vi "Main.vi"() -> ()   [LabVIEW 2013]
uses:
  <userlib>/KNR OS 3.0 LabVIEW Toolkit/Type Definition/Resource.ctl
panel:
  out "Numeric":i32
  out "LED List":bool[](array[boolean])
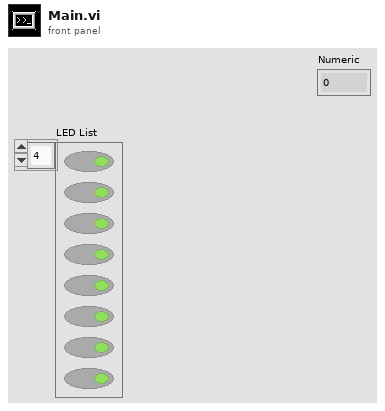
[diagram p1: front panel]
types:
  T1 = typedef "Resource.ctl" = enum16{"KNRm_DDRC", "KNRm_DDDD", "KNRm_DDDR", "KNRm_DDDC", "KNR"}
  T2 = typedef "KNR3 Reference.ctl" = cluster{"FPGA Session":refnum<class "FPGA Interface Base.lvclass">, "Resource":T1}
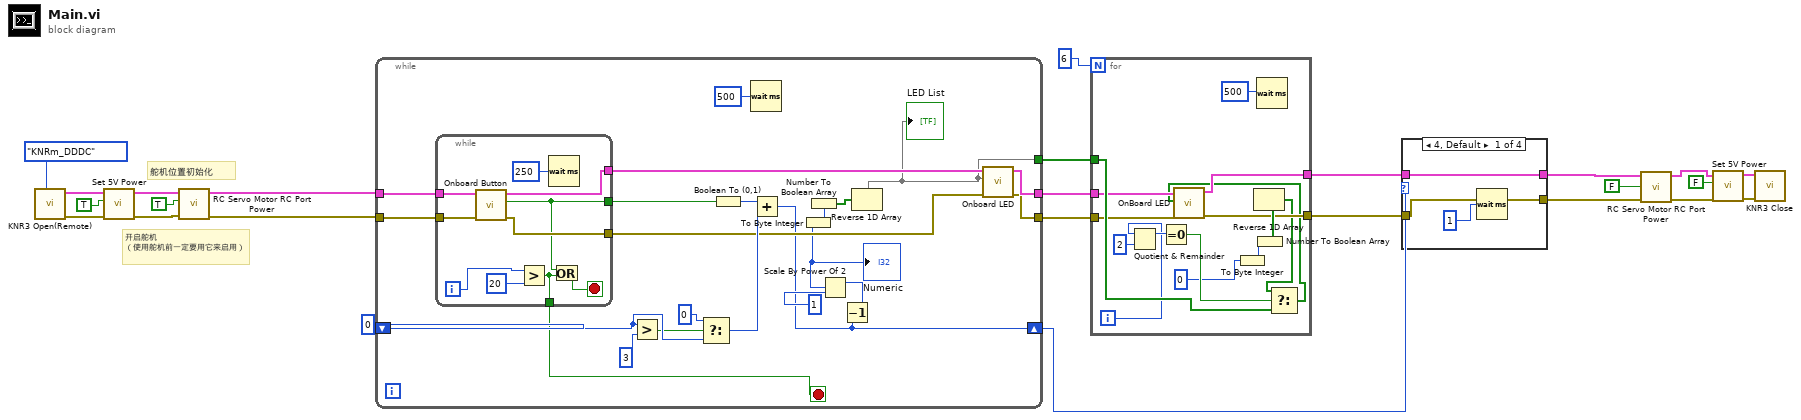
[diagram p0: block diagram]
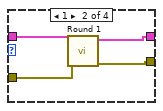
[diagram p2: hidden frame]
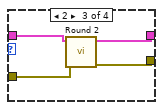
[diagram p3: hidden frame]
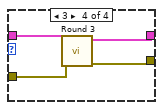
[diagram p4: hidden frame]
diagram:
  # "开启舵机\n（使用舵机前一定要用它来启用）"
  # "舵机位置初始化"
  n1 = call <userlib>:"KNR3 Open(Remote).vi"("Resource"=Resource."KNRm_DDDC") -> ("error out"=w22:errorcluster, "KNR out"=w23:T2)  [unwired: 9 in]
  n2 = call <userlib>:"Set 5V Power.vi"("error in (no error)"=w22, "5V Power(T)"=TRUE, "KNR in"=w23) -> ("error out"=w18:errorcluster, "KNR out"=w19:T2)  [unwired: 7 in]
  n3 = call <userlib>:"RC Servo Motor RC Port Power.vi"("error in (no error)"=w18, "RC Power(F)"=TRUE, "KNR in"=w19) -> ("error out"=w16:errorcluster, "KNR out"=w17:T2)  [unwired: 7 in]
  n4 = while {
    shift-right: [w30] -> w4
    shift-left: i8 0 -> [w46]
    tunnel: w17 -> [w42]
    tunnel: w16 -> [w41]
    tunnel: [w35] -> w3
    tunnel: [w34] -> w2
    tunnel: [w28] -> w1
    stop <- w27 stop-if-true
    n5 = while {
      tunnel: [w50] -> w44
      tunnel: w42 -> [w57]
      tunnel: w41 -> [w56]
      tunnel: [w54] -> w37
      tunnel: [w53] -> w36
      tunnel: [w48] -> w27
      i -> [w51]
      stop <- w49 stop-if-true
      n6 = call <userlib>:"Onboard Button.vi"("error in (no error)"=w56, "KNR in"=w57) -> ("error out"=w53:errorcluster, "value"=w50:bool, "KNR out"=w54:T2)  [unwired: 7 in]
      n7 = Greater?(x=w51, y=20) -> (0:w48:bool)
      n8 = Wait (ms)(milliseconds to wait=u32 250) -> ()  [unwired: 1 out]
      n9 = Or(x=w50, y=w48) -> (x .or. y?=w49:bool)
    }
    n10 = Greater?(x=w46, y=i8 3) -> (0:w39:bool)
    n11 = Select(t=0, s=w39, f=w46) -> (s? t:f=w45:i32)
    n12 = Boolean To (0,1)(Boolean=w44) -> (0, 1=w43:i16)
    n13 = Wait (ms)(milliseconds to wait=u32 500) -> ()  [unwired: 1 out]
    n14 = Add(x=w43, y=w45) -> (x+y=w30:i32)
    n15 = Decrement(x=w30) -> (x-1=w29:i32)
    n16 = Scale By Power Of 2(n=w29, x=1) -> (x*2^n=w32:i32)
    "Numeric" <- w32
    n17 = To Byte Integer(number=w32) -> (8bit integer=w31:i8)
    n18 = Number To Boolean Array(number=w31) -> (Boolean array=w38:bool[])
    n19 = Reverse 1D Array(array=w38) -> (reversed array=w28:bool[])
    "LED List" <- w28
    n20 = call <userlib>:"Onboard LED.vi"("error in (no error)"=w36, "LED List"=w28, "KNR in"=w37) -> ("error out"=w34:errorcluster, "KNR out"=w35:T2)  [unwired: 7 in]
  }
  n21 = for {
    N: i8 6 -> [_]
    tunnel: w1 -> [w70]
    tunnel: w3 -> [w66]
    tunnel: w2 -> [w65]
    tunnel: [w63] -> w7
    tunnel: [w62] -> w5
    i -> [w64]
    n22 = Quotient & Remainder(x=w64, y=i8 2) -> (x-y*floor(x/y)=w69:i32)  [unwired: 1 out]
    n23 = Equal To 0?(x=w69) -> (x = 0?=w68:bool)
    n24 = To Byte Integer(number=0) -> (8bit integer=w61:i8)
    n25 = Number To Boolean Array(number=w61) -> (Boolean array=w67:bool[])
    n26 = Reverse 1D Array(array=w67) -> (reversed array=w59:bool[])
    n27 = Wait (ms)(milliseconds to wait=500) -> ()  [unwired: 1 out]
    n28 = Select(t=w59, s=w68, f=w70) -> (s? t:f=w58:bool[])
    n29 = call <userlib>:"OnBoard LED.vi"("error in (no error)"=w65, "LED List"=w58, "KNR in"=w66) -> ("error out"=w62:errorcluster, "KNR out"=w63:T2)  [unwired: 7 in]
  }
  n30 = case shown="4, Default" w4 {
    tunnel: [w75 w77 w81 w86] -> w8
    tunnel: w7 -> [w75 w79 w83 w87]
    tunnel: [w74 w76 w80 w85] -> w6
    tunnel: w5 -> [w74 w78 w82 w84]
    frame 4, Default {
      n31 = Wait (ms)(milliseconds to wait=1) -> ()  [unwired: 1 out]
    }
    frame 1 {
      n32 = call "Round 1.vi"("error in (no error)"=w78, "KNR in"=w79) -> ("error out"=w76:errorcluster, "KNR out"=w77:T2)  [unwired: 8 in]
    }
    frame 2 {
      n33 = call "Round 2.vi"("error in (no error)"=w82, "KNR in"=w83) -> ("error out"=w80:errorcluster, "KNR out"=w81:T2)  [unwired: 8 in]
    }
    frame 3 {
      n34 = call "Round 3.vi"("error in (no error)"=w84, "KNR in"=w87) -> ("error out"=w85:errorcluster, "KNR out"=w86:T2)  [unwired: 8 in]
    }
  }
  n35 = call <userlib>:"RC Servo Motor RC Port Power.vi"("error in (no error)"=w6, "RC Power(F)"=FALSE, "KNR in"=w8) -> ("error out"=w9:errorcluster, "KNR out"=w10:T2)  [unwired: 7 in]
  n36 = call <userlib>:"Set 5V Power.vi"("error in (no error)"=w9, "5V Power(T)"=FALSE, "KNR in"=w10) -> ("error out"=w13:errorcluster, "KNR out"=w12:T2)  [unwired: 7 in]
  n37 = call <userlib>:"KNR3 Close.vi"("error in (no error)"=w13, "KNR in"=w12) -> ()  [unwired: 9 in, 1 out]
